vi "ReadTable.vi"(11 "HtmlString":string) -> (0 "Big5Text":string, 1 "ReleaseTime":string, 2 "tbodyData":string[][](array[string]), 3 "theadHead":string[](array[string]))   [LabVIEW 2013]
uses:
  <vilib>/regexp/Match Regular Expression.xnode
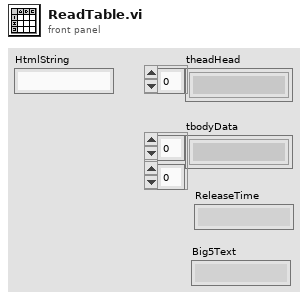
[diagram p1: front panel]
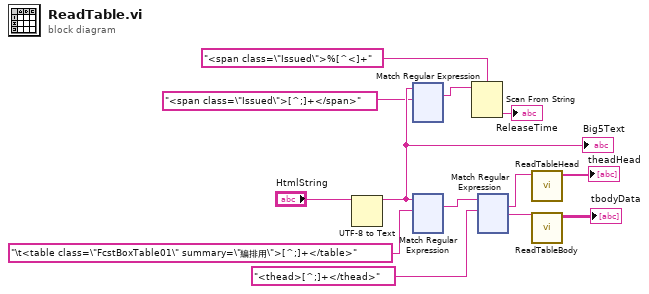
[diagram p0: block diagram]
diagram:
  n1 = UTF-8 to Text(11:"HtmlString") -> (3:w5:string)  [unwired: 1 in, 1 out]
  "Big5Text" <- w5
  n2 = xnode "Match Regular Expression"("input string"=w5, "regular expression"="<span class=\"Issued\">[^;]+</span>" ("body")) -> ("whole match"=w3:string)  [unwired: 4 in, 4 out]
  n3 = xnode "Match Regular Expression"("input string"=w5, "regular expression"="\t<table class=\"FcstBoxTable01\" summary=\"編排用\">[^;]+</table>" ("body")) -> ("whole match"=w9:string)  [unwired: 4 in, 4 out]
  n4 = Scan From String(format string="<span class=\"Issued\">%[^<]+" ("body"), input string=w3) -> (output 1=→"ReleaseTime":string)  [unwired: 3 in, 3 out]
  n5 = xnode "Match Regular Expression"("input string"=w9, "regular expression"="<thead>[^;]+</thead>" ("body")) -> ("whole match"=w10:string, "after match"=w12:string)  [unwired: 4 in, 3 out]
  n6 = call "ReadTableHead.vi"("theadString"=w10) -> ("theadData"=→"theadHead":string[])  [unwired: 10 in]
  n7 = call "ReadTableBody.vi"("tbodyString"=w12) -> ("tbodyData"=→"tbodyData":string[][])  [unwired: 10 in]
